vi "GamePadHacked.vi"(8 "error in (no error)":errorcluster, 11 "Refnum in":refnum<k1>) -> (0 "error out":errorcluster, 1 "Gamepad Output":T2, 2 "Control Cluster":T1 {"Yaw Speed" min=-1 max=1 step=0.01; "Vertical Speed" min=-1 max=1 step=0.01; "Pitch" min=-1 max=1 step=0.01; "Roll" min=-1 max=1 step=0.1}, 3 "Refnum out":refnum<k1>)   [LabVIEW 2014]
uses:
  <vilib>/Utility/inputDevices.llb/joystickAcquire.vi
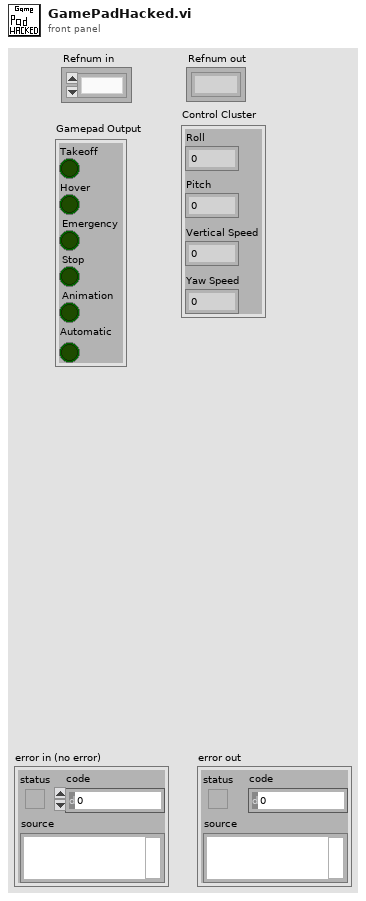
[diagram p1: front panel]
types:
  T1 = cluster{"Roll":sgl, "Pitch":sgl, "Vertical Speed":sgl, "Yaw Speed":sgl}
  T2 = cluster{"Takeoff":bool, "Hover":bool, "Emergency":bool, "Stop":bool, "Animation":bool, "Automatic":bool}
  T3 = cluster{"X axis":i32, "Y axis":i32, "Z axis":i32, "X axis rotation":i32, "Y axis rotation":i32, "Z axis rotation":i32, "U axis":i32, "V axis":i32}
  T4 = cluster{"button 1":bool, "button 2":bool, "button 3":bool, "button 4":bool, "button 5":bool, "button 6":bool, "button 7":bool, "button 8":bool, "button 9":bool, "button 10":bool, "button 11":bool, "button 12":bool, "button 13":bool, "button 14":bool, "button 15":bool, "button 16":bool, "button 17":bool, "button 18":bool, "button 19":bool, "button 20":bool, "button 21":bool, "button 22":bool, "button 23":bool, "button 24":bool, "button 25":bool, "button 26":bool, "button 27":bool, "button 28":bool, "button 29":bool, "button 30":bool, "button 31":bool, "button 32":bool}
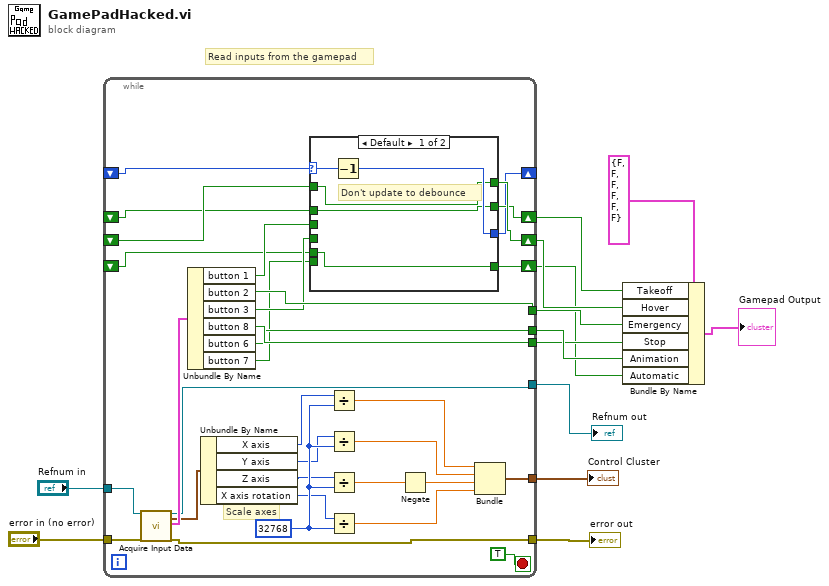
[diagram p0: block diagram]
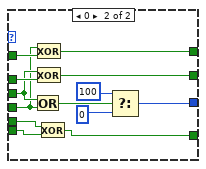
[diagram p2: hidden frame]
diagram:
  # "Read inputs from the gamepad"
  n1 = while {
    tunnel: [w45] -> w4
    tunnel: [w39] -> w8
    tunnel: [w34] -> w7
    tunnel: [w33] -> w13
    tunnel: "error in (no error)" -> [w32]
    tunnel: "Refnum in" -> [w31]
    tunnel: [w23] -> w10
    shift-right: [w41] -> w9
    shift-left: _ -> [w36]
    shift-right: [w40] -> w5
    shift-left: _ -> [w35]
    shift-right: [w18] -> _
    shift-left: _ -> [w19]
    tunnel: [w17] -> w6
    shift-right: [w15] -> w1
    shift-left: _ -> [w14]
    stop <- TRUE stop-if-true
    w30 = 32768
    # "Scale axes"
    n2 = call-poly <vilib>:"Acquire Input Data.vi"("device ID"=w31, "error in (no error)"=w32) -> ("device ID"=w23:refnum<k1>, "axis info"=w24:T3, "button info"=w25:T4, "error out"=w33:errorcluster)  [unwired: 13 in, 1 out]
    n3 = Unbundle By Name(w25) -> ("button 1"=w21:bool, "button 2"=w39:bool, "button 3"=w20:bool, "button 8"=w45:bool, "button 6"=w17:bool, "button 7"=w16:bool)
    n4 = Unbundle By Name(w24) -> ("X axis"=w26:i32, "Y axis"=w27:i32, "Z axis"=w28:i32, "X axis rotation"=w29:i32)
    n5 = case shown="Default" w19 {
      selector: w19 -> [w50 _]
      tunnel: [w47 w63] -> w41
      tunnel: [w48 w60] -> w40
      tunnel: w36 -> [w47 w62]
      tunnel: w35 -> [w48 w61]
      tunnel: w21 -> [_ w59]
      tunnel: w20 -> [_ w58]
      tunnel: [w49 w54] -> w18
      tunnel: w16 -> [_ w53]
      tunnel: [w46 w52] -> w15
      tunnel: w14 -> [w46 w51]
      frame Default {
        # "Don't update to debounce"
        n6 = Decrement(x=w50) -> (x-1=w49:i32)
      }
      frame 0 {
        n7 = Or(x=w59, y=w58) -> (x .or. y?=w57:bool)
        n8 = Exclusive Or(1:w62, 2:w58) -> (0:w63:bool)
        n9 = Exclusive Or(1:w61, 2:w59) -> (0:w60:bool)
        n10 = Exclusive Or(1:w53, 2:w51) -> (0:w52:bool)
        n11 = Select(t=100, s=w57, f=0) -> (s? t:f=w54:i32)
      }
    }
    n12 = Divide(x=w26, y=w30) -> (x/y=w38:dbl)
    n13 = Divide(x=w27, y=w30) -> (x/y=w42:dbl)
    n14 = Divide(x=w28, y=w30) -> (x/y=w43:dbl)
    n15 = Divide(x=w29, y=w30) -> (x/y=w37:dbl)
    n16 = Negate(x=w43) -> (-x=w44:dbl)
    n17 = Bundle(w38, w42, w44, w37) -> (w34:cluster{dbl, dbl, dbl, dbl})  [unwired: 1 in]
  }
  "error out" <- w13
  "Refnum out" <- w10
  "Control Cluster" <- w7
  n18 = Bundle By Name(cluster=T2 {"Takeoff"=FALSE, "Hover"=FALSE, "Emergency"=FALSE, "Stop"=FALSE, "Animation"=FALSE, "Automatic"=FALSE} ("Gamepad Output  Hacked"), "Takeoff"=w5, "Hover"=w9, "Emergency"=w8, "Stop"=w4, "Animation"=w6, "Automatic"=w1) -> (→"Gamepad Output":T2)
